vi "Kick User.vi"(8 "error in (no error)":errorcluster, 10 "User":string, 11 "LV Chat Server in":refnum<class "LV Chat Server.lvclass">) -> (0 "error out":errorcluster, 3 "LV Chat Server out":refnum<class "LV Chat Server.lvclass">)   [LabVIEW 2020, in "LV Chat Server.lvclass"]
uses:
  LV Chat Server.lvclass
  LV Chat Server.lvclass/LV Chat Server.ctl
  Stream-Simple-Msg/Endpoint/Endpoint.lvclass
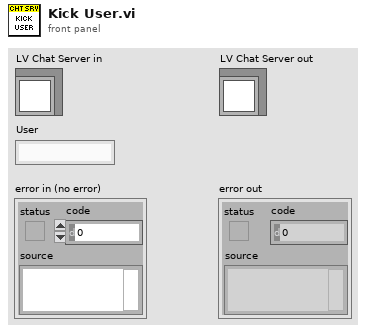
[diagram p1: front panel]
types:
  T1 = typedef "LV Chat Server.lvclass/Ref Data.ctl" = cluster{"Endpoint Map":map{string, T2}, "User Map":map{string, string}}
  T2 = typedef "LV Chat Server.lvclass/User.ctl" = cluster{"Name":string, "IP":string, "Connected At":dbl, "Endpoint":refnum<class "Endpoint.lvclass">}
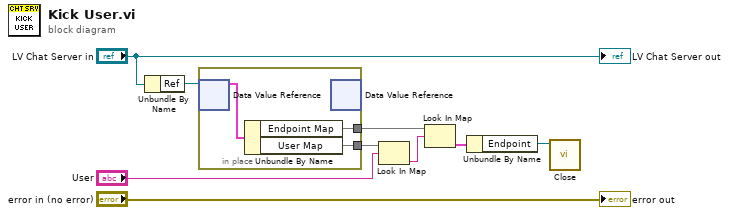
[diagram p0: block diagram]
diagram:
  n1 = Unbundle By Name("LV Chat Server in") -> ("Ref"=w8:refnum<data-value>)
  n2 = in-place {
    in-place-border: [w11] -> w6
    in-place-border: [w10] -> w7
    n3 = in-place-dvr #1(w8) -> (w12:T1)  [unwired: 1 out]
    n4 = Unbundle By Name(w12) -> ("Endpoint Map"=w11:map{string, T2}, "User Map"=w10:map{string, string})
    n5 = in-place-dvr #1() -> ()  [unwired: 1 in, 2 out]
  }
  n6 = Look In Map(map=w7, key="User") -> (value=w5:string)  [unwired: 1 in, 1 out]
  n7 = Look In Map(map=w6, key=w5) -> (value=w4:T2)  [unwired: 1 in, 1 out]
  n8 = Unbundle By Name(w4) -> ("Endpoint"=w3:refnum<class "Endpoint.lvclass">)
  n9 = call "Close.vi"("Endpoint in"=w3) -> ()  [unwired: 10 in, 1 out]
  "error out" <- "error in (no error)"
  "LV Chat Server out" <- "LV Chat Server in"
